vi "Actor Core.vi"(8 "error in":errorcluster, 11 "Example View in":refnum<class "Example View 2.lvclass">) -> (0 "error out":errorcluster, 3 "Actor out":refnum<class "Actor.lvclass">)   [LabVIEW 2023, in "Example MVC Actors.lvlib" / "Example View 2.lvlib" / "Example View 2.lvclass"]
doc: "(<B>Filename</B>: Actor Framework.lvlib:Actor.lvclass:Actor Core.vi)\n\nReceives messages to the actor, reacts to them, and initiates any error handling that may shut the actor down.\n\nDescendant classes may override this VI to append parallel tasks for the actor to complete while it handles messages. Overrides use the Call Parent Method node."
uses:
  Example View 2.lvclass
  C:/Program Files/National Instruments/LabVIEW 2023/vi.lib/ActorFramework/Actor/Actor.lvclass
  C:/Projects/Shared Libraries/Event Actors/View/View.lvclass
  <vilib>/ActorFramework/Actor/Actor.lvclass
  Example View 2.lvclass/Example View 2.ctl
  <vilib>/ActorFramework/Actor/Actor.lvclass/Actor.ctl
  <vilib>/ActorFramework/Message Enqueuer/Message Enqueuer.lvclass/Message Enqueuer.ctl
  View/View.lvclass/View.ctl
  Example Events/Boolean Event.lvclass
  C:/Projects/Shared Libraries/Event Actors/Event Data Types/Event Boolean/Event Boolean.lvclass
  C:/Projects/Shared Libraries/Event Actors/Event/Event.lvclass
  Event/Event.lvclass/Event.ctl
  Example View Messages/Example View 2/Update Boolean Event Msg/Update Boolean Event Msg.lvclass
  C:/Projects/Shared Libraries/Event Actors/Event Handlers/Abstract Event Message for View/Abstract Event Message for View.lvclass
  View/properties/Read Name.vi
  <vilib>/ActorFramework/Message Enqueuer/Init from Existing Queue.vi
  <vilib>/ActorFramework/Message Enqueuer/Message Enqueuer.lvclass
  View/View.lvclass
  View Messages/Generate and Broadcast Event Msg/Generate and Broadcast Event Msg.lvclass
  Event/Event.lvclass
  View Messages/Unregister Event Msg/Unregister Event Msg.lvclass
  View Messages/Register Event Msg/Register Event Msg.lvclass
panel:
  in  "Get Last Broadcast Event":bool=TRUE
  in  "Registered for Boolean":bool
  out "View Name":string
  in  "Boolean":bool
  # "This View is not automatically launched by the Controller but  launched manually from the Controller GUI. This View doesn't register any event upon initilaization, but allows for registration of the Boolean event from this GUI by calling the Controller's method \"Register by Name.vi\" with the option \"Get Last Broadcast Event (F)\"  set to the corresponding GUI chackbox. This means that, if the Boolean event was previously fired either by the Controller or by one of the Views, when this Event is registered the Controller will generate the latest broadcast value of such event to this View. \n\nInstrunctions:\n1. Launch the example\n2. From the Controller launch this view\n3. From one of the Views set the Boolean controller to true\n4. Register to the boolean event form this GUI\n5. Observe in this VIew that the Boolean control is set to true\n6. Repeat the same forcedure omitting step 2. and observe that the Boolean controller  is set to false"
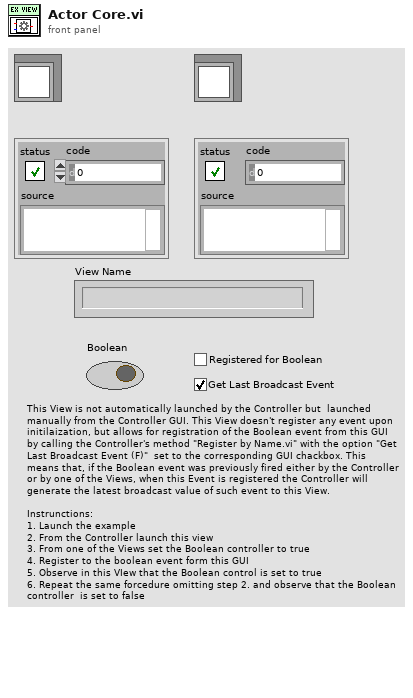
[diagram p1: front panel]
types:
  T1 = enum8{"Enabled", "Disabled", "Disabled and Grayed Out"}
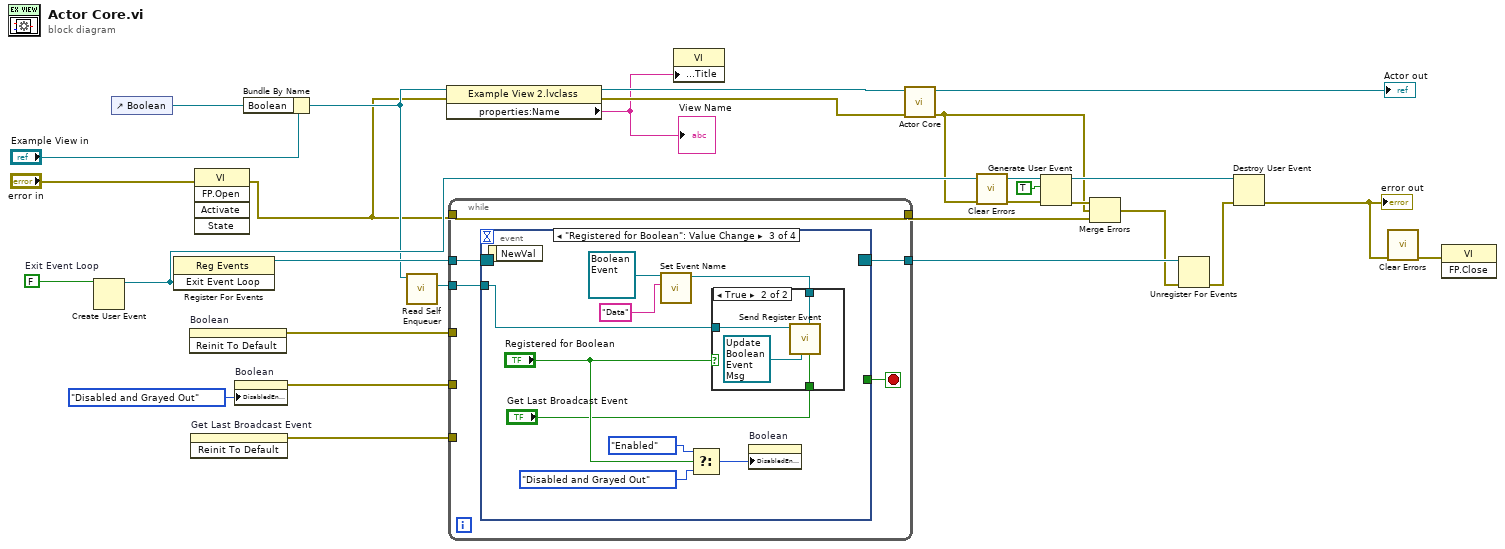
[diagram p0: block diagram]
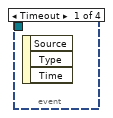
[diagram p2: hidden frame]
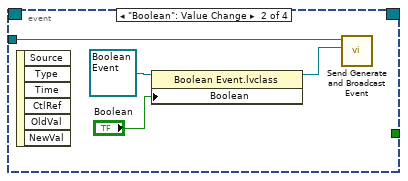
[diagram p3: hidden frame]
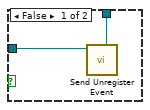
[diagram p4: hidden frame]
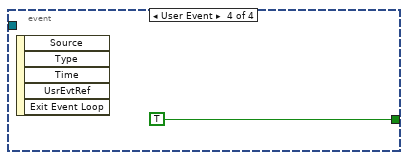
[diagram p5: hidden frame]
diagram:
  w23 = FALSE  # Exit Event Loop
  n1 = Create User Event(user event datatype=w23) -> (user event=w20:refnum<user-event>)  [unwired: 1 in, 1 out]
  n2 = control-ref of="Boolean"() -> (w26:refnum<vi>)
  n3 = register-events(w20) -> (reference out=w22:refnum<event-registration>)  [unwired: 2 in, 1 out]
  n4 = invoke on="Boolean" class="Bool (strict)" method="Reinit To Default"() -> (error out=w4:errorcluster)  [unwired: 3 in, 2 out]
  n5 = invoke on="Get Last Broadcast Event" class="Bool (strict)" method="Reinit To Default"() -> (error out=w1:errorcluster)  [unwired: 3 in, 2 out]
  n6 = invoke class="VI" method="FP.Open"(error in="error in") -> (error out=w7:errorcluster)  [unwired: 4 in, 4 out]
  n7 = property on="Boolean" class="Bool (strict)"("DisabledEnum"=T1."Disabled and Grayed Out" ("Disabled")) -> (error out=w2:errorcluster)  [unwired: 2 in, 1 out]
  n8 = Bundle By Name(cluster="Example View in", "Boolean"=w26) -> (w15:refnum<class "Example View 2.lvclass">)
  n9 = call <vilib>:"Read Self Enqueuer.vi"("Actor"=w15) -> ("Self Enqueuer"=w24:refnum<class "Message Enqueuer.lvclass">)  [unwired: 10 in]
  n10 = property class="Example View 2.lvclass"(reference=w15, error in=w7) -> (reference out=w8:refnum<class "Example View 2.lvclass">, error out=w6:errorcluster, "properties:Name"=w5:string)
  "View Name" <- w5
  n11 = while {
    tunnel: w24 -> [w33]
    tunnel: w22 -> [w32]
    tunnel: w7 -> [w31]
    tunnel: [w31] -> w14
    tunnel: [w30] -> w18
    tunnel: w4 -> [_]
    tunnel: w2 -> [_]
    tunnel: w1 -> [_]
    stop <- w29 stop-if-true
    n12 = event shown="[2] \"Registered for Boolean\": Value Change" {
      selector: w32 -> [_ _ _ _]
      dyn-events: [_ _ _ _] -> w30
      timeout: _ -> [_ _ _ _]
      tunnel: w33 -> [_ w37 w43 _]
      tunnel: [_ _ _ TRUE] -> w29
      event Timeout {
        n13 = event-data() -> ()  [unwired: 1 in, 3 out]
      }
      event "Boolean": Value Change {
        n14 = event-data() -> ()  [unwired: 1 in, 6 out]
        n15 = property class="Boolean Event.lvclass"(reference=refnum<class "Boolean Event.lvclass"> refnum ("Example Source.lvlib:Boolean Event.lvclass"), "Boolean"="Boolean") -> (reference out=w34:refnum<class "Boolean Event.lvclass">)  [unwired: 1 in, 1 out]
        n16 = call "Send Generate and Broadcast Event.vi"("Event Data"=w34, "Message Enqueuer in"=w37) -> ()  [unwired: 8 in, 2 out]
      }
      event "Registered for Boolean": Value Change {
        n17 = event-data() -> ()  [unwired: 1 in, 1 out]
        n18 = call "Set Event Name.vi"("Name (Generic)"="Data", "Event In"=refnum<class "Boolean Event.lvclass"> refnum ("Example Source.lvlib:Boolean Event.lvclass")) -> ("Event Out"=w46:refnum<class "Boolean Event.lvclass">)  [unwired: 9 in]
        n19 = Select(t=T1."Enabled" ("Disabled"), s="Registered for Boolean", f=T1."Disabled and Grayed Out" ("Disabled")) -> (s? t:f=w39:T1)
        n20 = case shown="True" "Registered for Boolean" {
          tunnel: w46 -> [w48 w52]
          tunnel: w43 -> [w47 w51]
          tunnel: "Get Last Broadcast Event" -> [_ w49]
          frame False {
            n21 = call "Send Unregister Event.vi"("Event"=w48, "Message Enqueuer in"=w47) -> ()  [unwired: 8 in, 2 out]
          }
          frame True {
            n22 = call "Send Register Event.vi"("Get Last Broadcast Event (F)"=w49, "Event"=w52, "Event Handler"=refnum<class "Update Boolean Event Msg.lvclass"> refnum ("Example Event Actors.lvlib:Example View Actor 2.lvlib:Update Boolean Event Msg.lvclass"), "Message Enqueuer in"=w51) -> ()  [unwired: 6 in, 2 out]
          }
        }
        n23 = property on="Boolean" class="Bool (strict)"("DisabledEnum"=w39) -> ()  [unwired: 2 in, 2 out]
      }
      event User Event {
        n24 = event-data() -> ()  [unwired: 1 in, 5 out]
      }
    }
  }
  n25 = property class="VI"("Front Panel.Title"=w5) -> ()  [unwired: 2 in, 2 out]
  n26 = call-parent "Actor Core.vi"("error in"=w6, "Actor in"=w8) -> ("error out"=w10:errorcluster, "Actor out"=→"Actor out":refnum<class "Actor.lvclass">)  [unwired: 8 in]
  n27 = call <vilib>:"Clear Errors.vi"("error in (no error)"=w10) -> ("error out"=w9:errorcluster)  [unwired: 5 in, 1 out]
  n28 = Generate User Event(user event=w20, event data cluster=TRUE ("event data"), error in=w9) -> (user event out=w19:refnum<user-event>, error out=w21:errorcluster)  [unwired: 1 in]
  n29 = Merge Errors(w21, w10, w14) -> (w11:errorcluster)
  n30 = Unregister For Events(event registration refnum=w18, error in=w11) -> (error out=w17:errorcluster)
  n31 = Destroy User Event(user event=w19, error in=w17) -> (error out=w12:errorcluster)
  "error out" <- w12
  n32 = call <vilib>:"Clear Errors.vi"("error in (no error)"=w12) -> ("error out"=w13:errorcluster)  [unwired: 5 in, 1 out]
  n33 = invoke class="VI" method="FP.Close"(error in=w13) -> ()  [unwired: 2 in, 3 out]
